vi "Restart System.vi"(8 "error in":errorcluster, 11 "tCRD in":refnum<class "Open Path CRD.lvclass">) -> (0 "error out":errorcluster, 3 "tCRD out":refnum<class "Open Path CRD.lvclass">)   [LabVIEW 2015, in "Open Path CRD.lvclass"]
doc: "If a restart has been requested, then we will grab a single record and check that record for a discontinuity. If one exists, retrieve the number of elements from the CRD Data buffer up to the location of the discontinuity. Reset the Restart Requested? flag."
uses:
  Open Path CRD.lvclass
  Reusable/Instrument/Instrument.lvclass/Instrument.ctl
  Open Path CRD.lvclass/Open Path CRD.ctl
  Reusable/Instrument/Write Restart Requested_.vi
  Reusable/Instrument/Read Restart Requested_.vi
  Accessors/Read FPGA Ref.vi
  Accessors/Read SamplesPerRep.vi
  Reusable/Instrument/Read Log Session.vi
  <vilib>/Utility/error.llb/Error Cluster From Error Code.vi
  <vilib>/rvi/errors/niLvFpgaAdjustHostInterfaceError.vi
  Open Path FPGA Ref.ctl
  <userlib>/_Session Fwk/Session - Root.lvclass
  <vilib>/rvi/interface/nirviMethod/nirviMethod.xnode
  FPGA Bitfiles/80MHz_server.lvbitx
  <vilib>/rvi/errors/niLvFpgaMergeErrorWithErrorCode.vi
  Reusable/Session Log/System Log.lvclass
  <vilib>/FPGAPlugInAG/sbRIO-9637/niLvFpga_ReadFifo_sbRIO-9637.vi
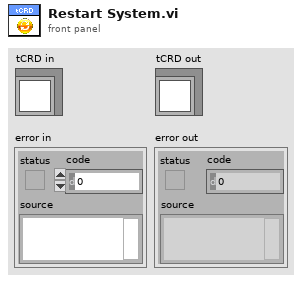
[diagram p1: front panel]
types:
  T1 = typedef "Open Path CRD.lvclass/Open Path FPGA Ref.ctl" = refnum<k20>
  T2 = typedef "Session - Root.lvclass/Session Handle.ctl" = refnum<data-value>
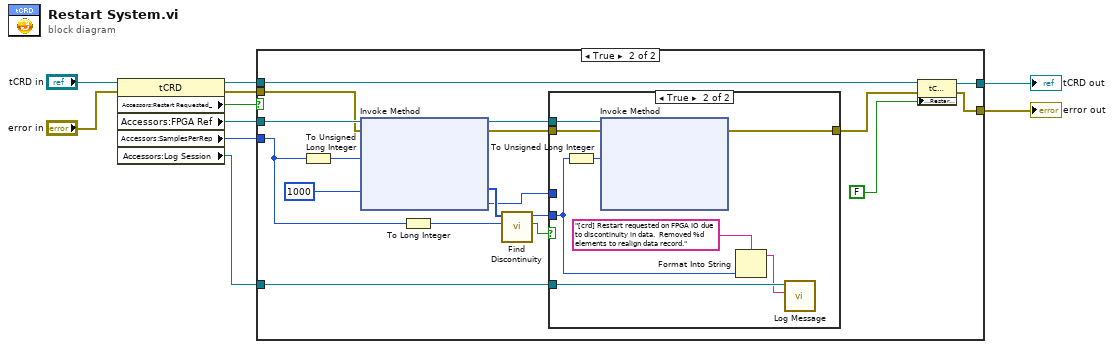
[diagram p0: block diagram]
diagram:
  n1 = property class="tCRD"(reference="tCRD in", error in="error in") -> (reference out=w3:refnum<class "Open Path CRD.lvclass">, error out=w5:errorcluster, "Accessors:Restart Requested_"=w8:bool, "Accessors:FPGA Ref"=w7:T1, "Accessors:SamplesPerRep"=w6:u16, "Accessors:Log Session"=w1:T2)
  n2 = case shown="True" w8 {
    tunnel: w7 -> [_ w30]
    tunnel: w6 -> [_ w16]
    tunnel: w5 -> [w12 w23]
    tunnel: [w12 w18] -> w4
    tunnel: w3 -> [w11 w22]
    tunnel: [w11 w20] -> w2
    tunnel: w1 -> [_ w14]
    frame False {
    }
    frame True {
      n3 = To Unsigned Long Integer(number=w16) -> (unsigned 32bit integer=w17:u32)
      n4 = xnode "Invoke Method"("FPGA VI Reference In"=w30, "error in"=w23, "Number of Elements"=w17, "Timeout (ms)"=1000) -> ("FPGA VI Reference Out"=w27:T1, "error out"=w24:errorcluster, "Data"=w28:i16[], "Elements Remaining"=w13:u32)
      n5 = To Long Integer(number=w16) -> (32bit integer=w15:i32)
      n6 = call "Find Discontinuity.vi"("Single Record"=w15, "Data"=w28) -> ("Discontinuity Detected"=w26:bool, "cIndex"=w25:i32)  [unwired: 8 in]
      n7 = case shown="True" w26 {
        tunnel: w27 -> [_ w39]
        tunnel: w25 -> [_ w33]
        tunnel: w24 -> [w31 w38]
        tunnel: [w31 w37] -> w19
        tunnel: w14 -> [_ w35]
        tunnel: w13 -> [_ _]
        frame False {
        }
        frame True {
          n8 = To Unsigned Long Integer(number=w33) -> (unsigned 32bit integer=w36:u32)
          n9 = xnode "Invoke Method"("FPGA VI Reference In"=w39, "error in"=w38, "Number of Elements"=w36) -> ("error out"=w37:errorcluster)  [unwired: 1 in, 3 out]
          n10 = Format Into String(format string="[crd] Restart requested on FPGA IO due to discontinuity in data.  Removed %d elements to realign data record." ("MSG In"), w33) -> (resulting string=w32:string)  [unwired: 2 in, 1 out]
          n11 = call "Log Message.vi"("MSG In"=w32, "session in"=w35) -> ()  [unwired: 8 in, 2 out]
        }
      }
      n12 = property class="tCRD"(reference=w22, error in=w19, "Accessors:Restart Requested_"=FALSE ("Restart Requested_")) -> (reference out=w20:refnum<class "Open Path CRD.lvclass">, error out=w18:errorcluster)
    }
  }
  "error out" <- w4
  "tCRD out" <- w2
